vi "extractTachometerData.vi"(8 "error in (no error)":errorcluster, 11 "Model in":refnum<class "Model.lvclass">) -> (0 "error out":errorcluster, 3 "Model out":refnum<class "Model.lvclass">)   [LabVIEW 2013, in "Model.lvclass"]
uses:
  Model.lvclass
  <userlib>/Common/ILC/ILCModelTypedefs/FinalDelimiter.ctl
  Model.lvclass/Model.ctl
  <userlib>/Common/ILC/ILCModelTypedefs/ILCModelTypedefs.lvlib
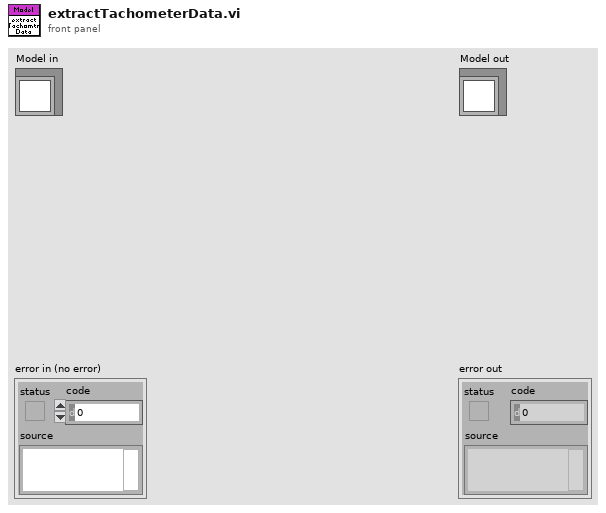
[diagram p1: front panel]
types:
  T1 = typedef "ILCCommon.lvlib/ILCModelTypedefs.lvlib/FinalDelimiter.ctl" = enum16{",", "<CR><LF>"}
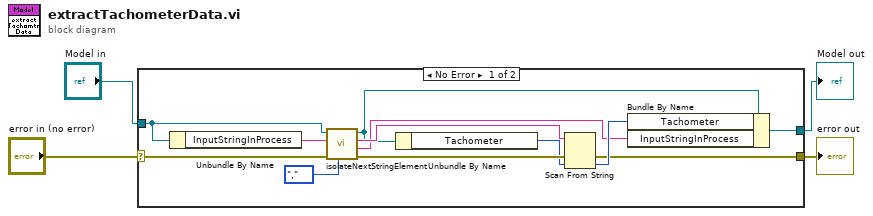
[diagram p0: block diagram]
diagram:
  n1 = case shown="No Error" "error in (no error)" {
    selector: "error in (no error)" -> [w10 w18]
    tunnel: [w9 w18] -> w3
    tunnel: [w11 w17] -> w1
    tunnel: "Model in" -> [w7 w17]
    frame No Error {
      n2 = Unbundle By Name(w7) -> ("InputStringInProcess"=w8:string)
      n3 = call "isolateNextStringElement.vi"("Final Delimiter"=FinalDelimiter.",", "error in (no error)"=w10, "inputString"=w8, "Model in"=w7) -> ("error out"=w15:errorcluster, "remainingString"=w5:string, "extractedSegment"=w16:string, "Model out"=w6:refnum<class "Model.lvclass">)  [unwired: 4 in]
      n4 = Unbundle By Name(w6) -> ("Tachometer"=w12:u16)
      n5 = Scan From String(input string=w16, error in=w15, default 1=w12) -> (error out=w9:errorcluster, output 1=w13:u16)  [unwired: 2 in, 2 out]
      n6 = Bundle By Name(cluster=w6, "Tachometer"=w13, "InputStringInProcess"=w5) -> (w11:refnum<class "Model.lvclass">)
    }
    frame Error {
    }
  }
  "error out" <- w3
  "Model out" <- w1
